vi "Martinas Aging Program v1.0.vi"() -> ()   [LabVIEW 2011]
panel:
  in  "stop":bool
  out "Table in useful format 2":T1(array[cluster])=[{"Label"="Cell 1", "Area (cm^2)"=0.15, "Position"=1, "Comment"="pedot on glass", "Scan Table"=array1000x2[2000 elements], "seconds since 1Jan1904"=timestamp(0 s since 1904-01-01), "t0"=0.0}, {"Label"="Cell 2", "Area (cm^2)"=0.12, "Position"=5, "Comment"="glass on glass", "Scan Table"=array1000x2[2000 elements], "seconds since 1Jan1904"=timestamp(0 s since 1904-01-01), "t0"=0.0}, {"Label"="Cell 3", "Area (cm^2)"=0.14, "Position"=3, "Comment"="gold on pedot", "Scan Table"=array1000x2[2000 elements], "seconds since 1Jan1904"=timestamp(0 s since 1904-01-01), "t0"=0.0}]
  in  "Total Number of Scans":i32=5
  in  "Interval (s)":i64=5
  out "Queue":string[][](table)
  in  "Cell Table":string[][](table)=[["Cell 1", "0.15", "1", "pedot on glass"], ["Cell 2", "0.12", "5", "glass on glass"], ["Cell 3", "0.14", "3", "gold on pedot"]]
  # "Label"
  # "Area"
  # "Position"
  # "Comment"
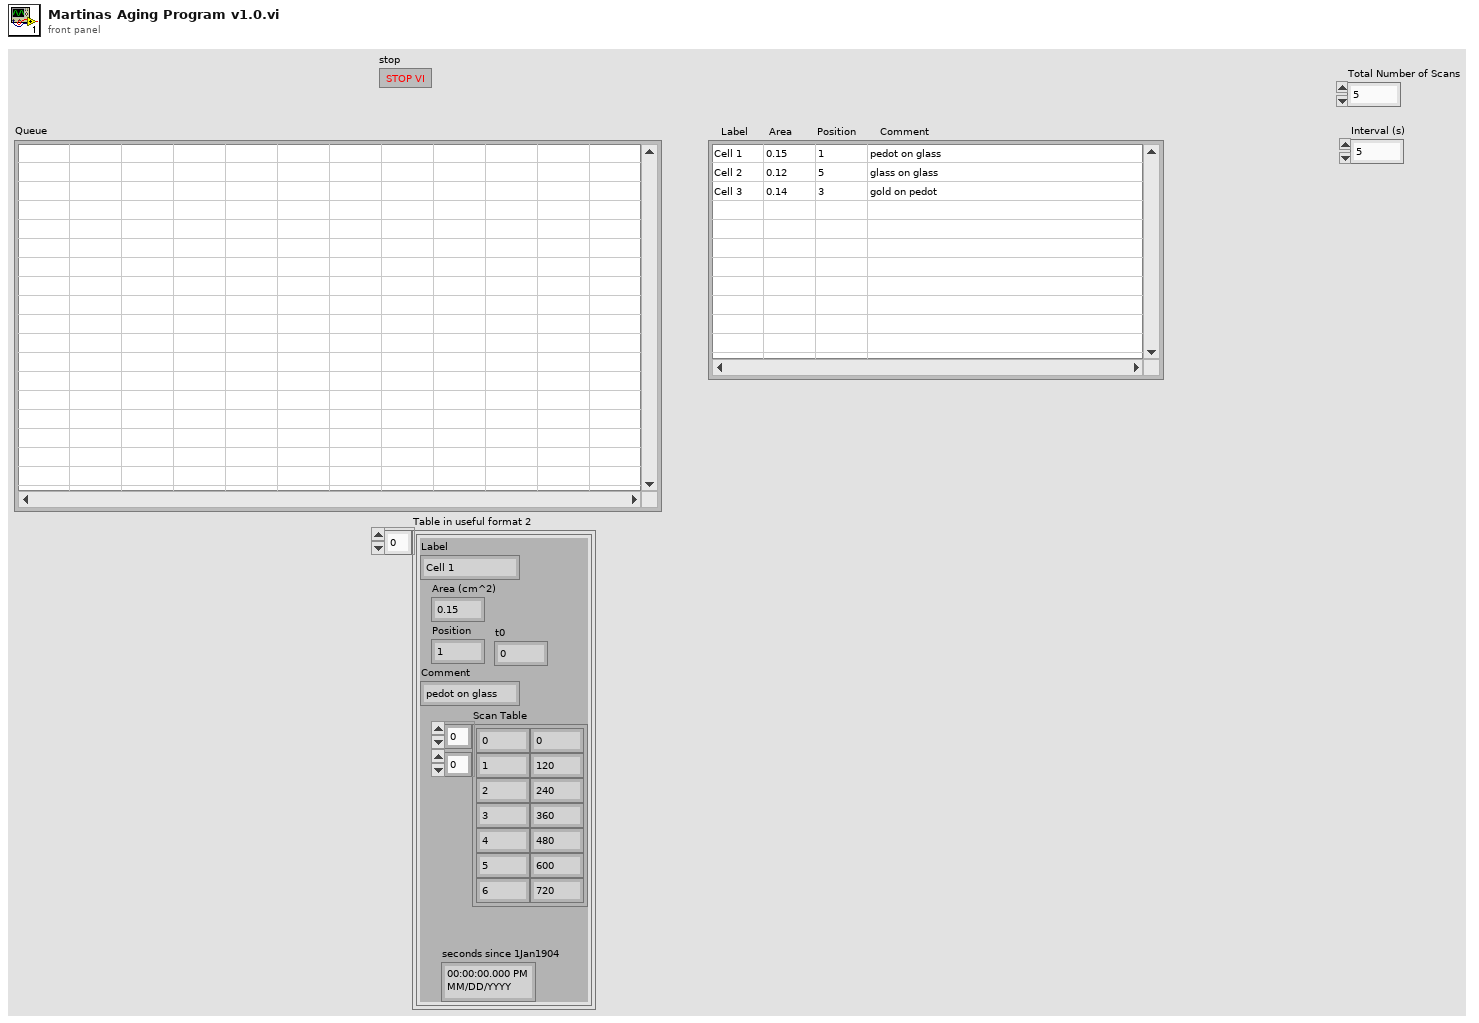
[diagram p1: front panel]
types:
  T1 = cluster{"Label":string, "Area (cm^2)":dbl, "Position":i32, "Comment":string, "Scan Table":dbl[][], "seconds since 1Jan1904":timestamp, "t0":dbl}[]
  T2 = cluster{"Label":string, "Area (cm^2)":dbl, "Position":i32, "Comment":string, "Scan Table":dbl[][], "seconds since 1Jan1904":timestamp, "t0":dbl}
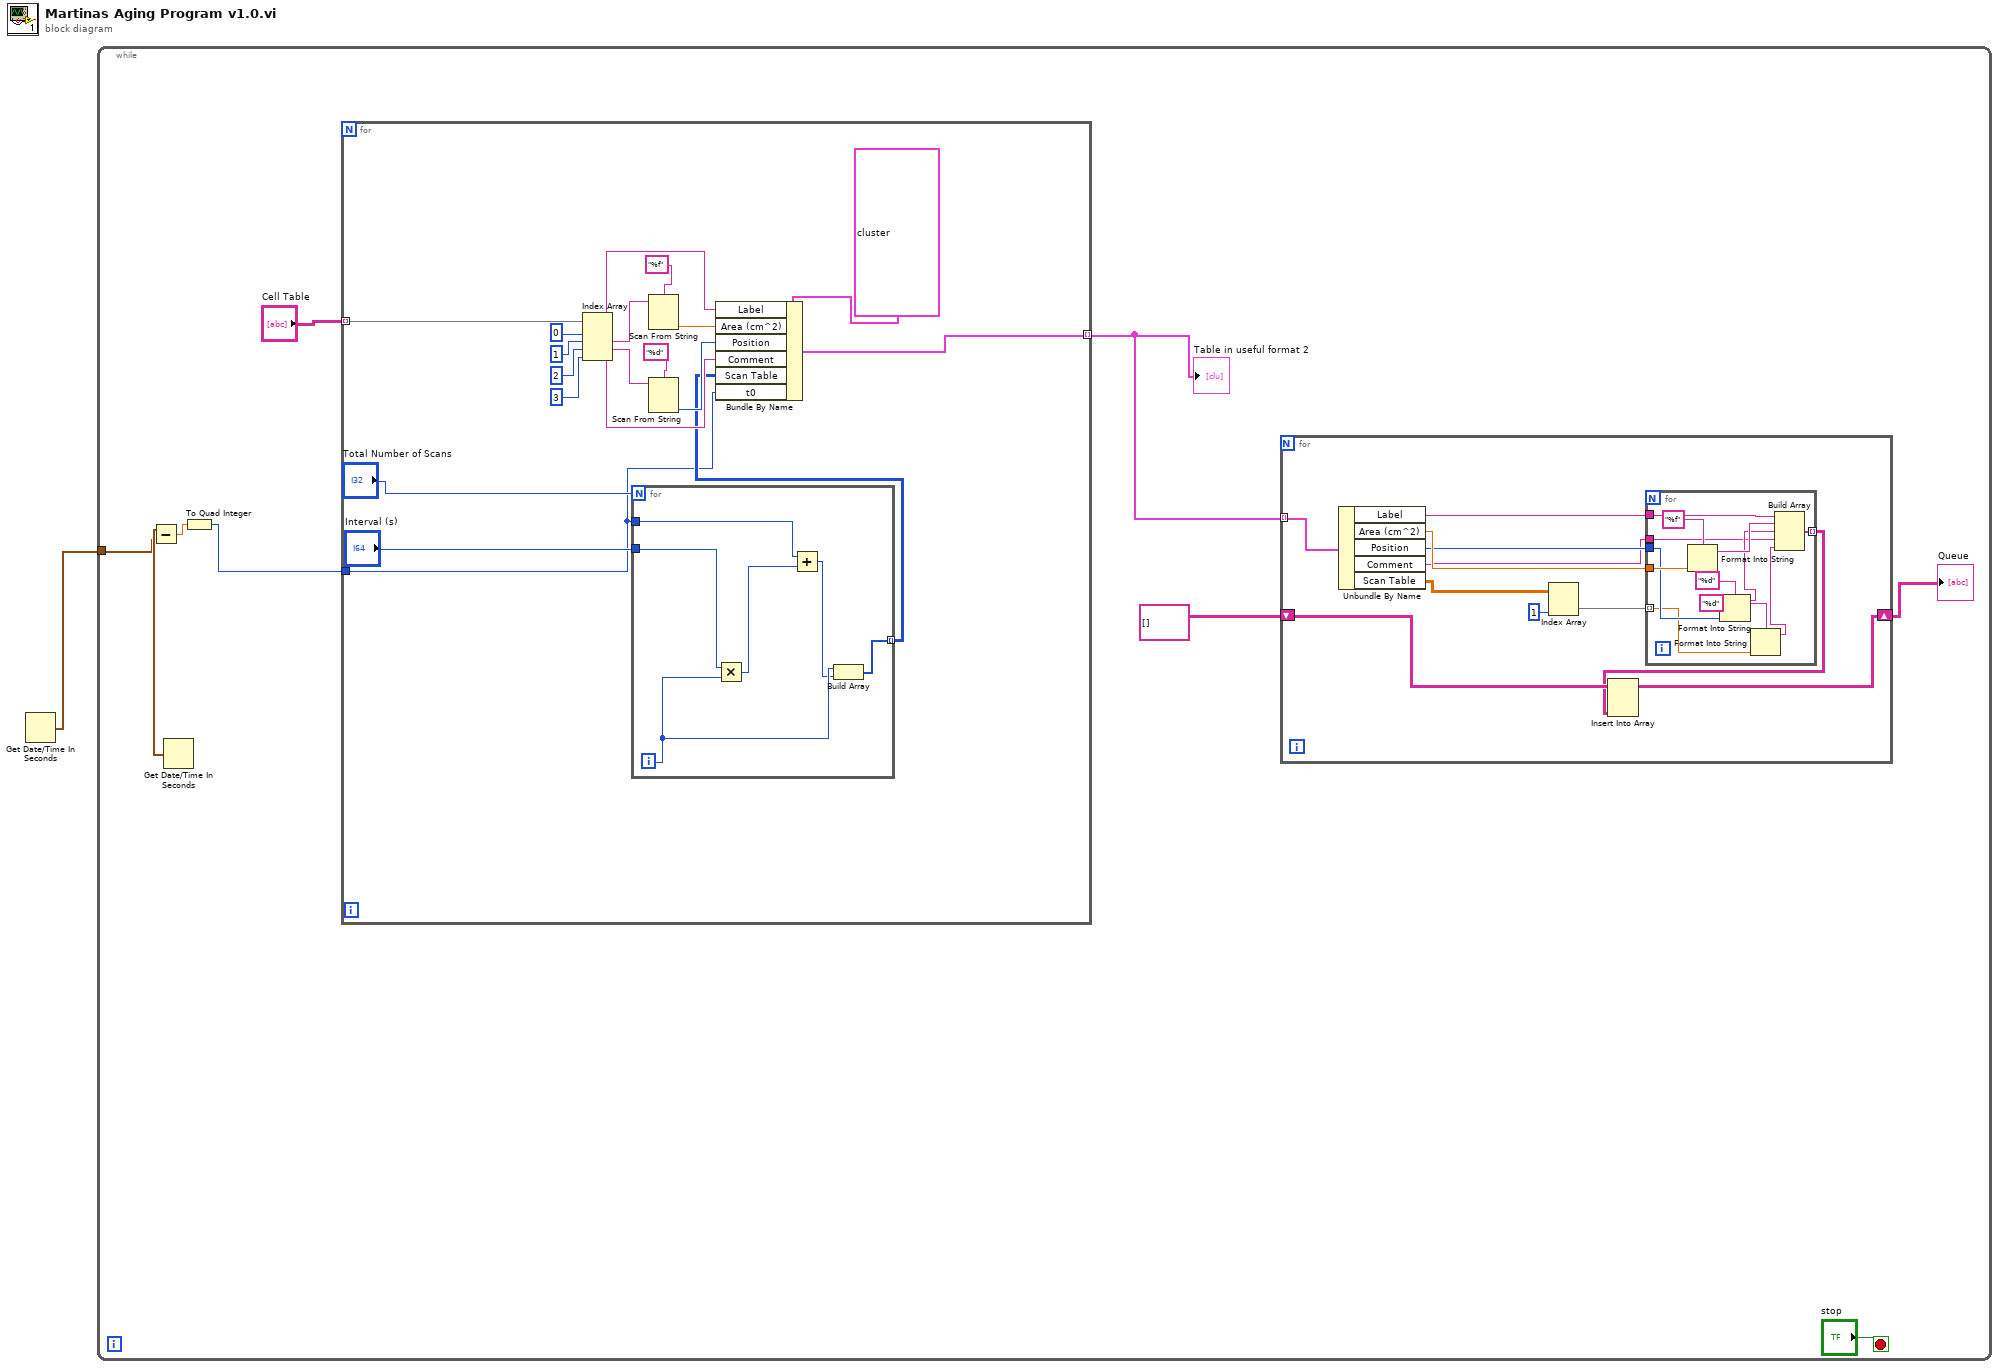
[diagram p0: block diagram]
diagram:
  n1 = Get Date/Time In Seconds() -> (seconds since 1Jan1904=w1:timestamp)
  n2 = while {
    tunnel: w1 -> [w7]
    stop <- "stop" stop-if-true
    n3 = Get Date/Time In Seconds() -> (seconds since 1Jan1904=w8:timestamp)
    n4 = Subtract(x=w8, y=w7) -> (x-y=w6:dbl)
    n5 = To Quad Integer(1:w6) -> (0:w5:i64)
    n6 = for {
      tunnel: "Cell Table" -> [w52] mode=indexing
      tunnel: [w39] -> w4 mode=indexing
      tunnel: w5 -> [w34]
      n7 = Index Array(array=w52, index #1=0 ("index"), index #2=1 ("index"), index #3=2 ("index"), index #4=3 ("index")) -> (element #1=w47:string, element #2=w45:string, element #3=w42:string, element #4=w46:string)
      n8 = for {
        N: "Total Number of Scans" -> [_]
        tunnel: "Interval (s)" -> [w58]
        tunnel: [w56] -> w36 mode=indexing
        tunnel: w34 -> [w54]
        i -> [w57]
        n9 = Multiply(x=w58, y=w57) -> (x*y=w55:i64)
        n10 = Add(x=w54, y=w55) -> (x+y=w53:i64)
        n11 = Build Array(w57, w53) -> (w56:i64[])
      }
      n12 = Scan From String(format string="%f", input string=w45) -> (output 1=w43:dbl)  [unwired: 3 in, 3 out]
      n13 = Scan From String(format string="%d", input string=w42) -> (output 1=w40:i32)  [unwired: 3 in, 3 out]
      n14 = Bundle By Name(cluster=T2 {"Label"="Cell 1", "Area (cm^2)"=0.15, "Position"=1, "Comment"="pedot on glass", "Scan Table"=array1000x2[2000 elements], "seconds since 1Jan1904"=timestamp(0 s since 1904-01-01), "t0"=0.0} ("Cluster 2"), "Label"=w47, "Area (cm^2)"=w43, "Position"=w40, "Comment"=w46, "Scan Table"=w36, "t0"=w34) -> (w39:T2)
    }
    "Table in useful format 2" <- w4
    n15 = for {
      tunnel: w4 -> [w21] mode=indexing
      shift-right: [w11] -> w2
      shift-left: string[][] [] ("Queue") -> [w13]
      n16 = Unbundle By Name(w21) -> ("Label"=w17:string, "Area (cm^2)"=w16:dbl, "Position"=w15:i32, "Comment"=w14:string, "Scan Table"=w20:dbl[][])
      n17 = Index Array(array=w20, index (col)=1 ("disabled index (col)")) -> (element=w18:dbl[])  [unwired: 1 in]
      n18 = for {
        tunnel: w18 -> [w24] mode=indexing
        tunnel: w17 -> [w33]
        tunnel: w16 -> [w32]
        tunnel: w15 -> [w28]
        tunnel: w14 -> [w26]
        tunnel: [w22] -> w12 mode=indexing
        n19 = Format Into String(format string="%f", w32) -> (resulting string=w30:string)  [unwired: 2 in, 1 out]
        n20 = Format Into String(format string="%d", w28) -> (resulting string=w27:string)  [unwired: 2 in, 1 out]
        n21 = Format Into String(format string="%d", w24) -> (resulting string=w23:string)  [unwired: 2 in, 1 out]
        n22 = Build Array(w33, w30, w27, w26, w23) -> (w22:string[])
      }
      n23 = Insert Into Array(array=w13, new element=w12) -> (w11:string[][])  [unwired: 2 in]
    }
    "Queue" <- w2
  }
